vi "DriveWaitForButton.vi"(2 "Parameter String":string, 3 "Reinit":bool) -> (0 "Error Out":errorcluster, 1 "Increment":bool)   [LabVIEW 2019]
doc: "This VI pauses the drive sequencer until the driver presses the \"advance system check\" button on the joystick, the joystick will rumble while waiting for the button."
uses:
  dscommands.vi
  dsdata.vi
  autoninfo.vi
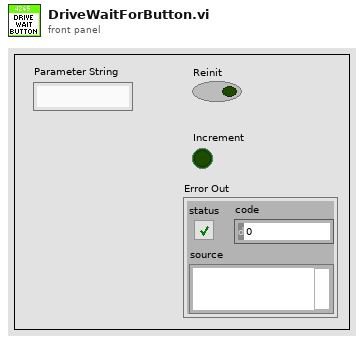
[diagram p1: front panel]
types:
  T1 = enum16{"Center", "North", "NorthWest", "West", "SouthWest", "South", "SouthEast", "East", "NorthEast"}
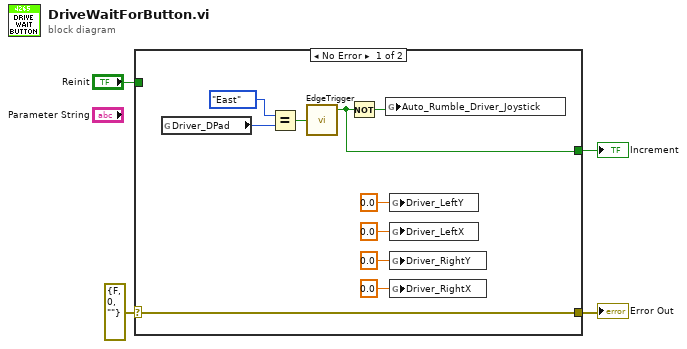
[diagram p0: block diagram]
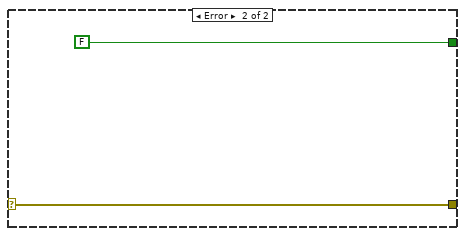
[diagram p2: hidden frame]
diagram:
  n1 = case shown="No Error" errorcluster {"status"=FALSE, "code"=0, "source"=""} ("error IO") {
    selector: errorcluster {"status"=FALSE, "code"=0, "source"=""} ("error IO") -> [w10 w16]
    tunnel: [w5 FALSE] -> w4
    tunnel: "Reinit" -> [_ _]
    tunnel: [w10 w16] -> w2
    frame No Error {
      n2 = global read "dsdata.vi" "Driver_DPad"() -> (w9:T1)
      n3 = Equal?(x=T1."East" ("Driver_DPad"), y=w9) -> (x = y?=w7:bool)
      n4 = call "EdgeTrigger.vi"("Input Signal"=w7) -> ("Rising Edge Trigger"=w5:bool)  [unwired: 2 out]
      n5 = Not(x=w5) -> (.not. x?=w8:bool)
      n6 = global write "autoninfo.vi" "Auto_Rumble_Driver_Joystick"(w8) -> ()
      n7 = global write "dscommands.vi" "Driver_LeftY"(0.0 ("Driver_LeftY")) -> ()
      n8 = global write "dscommands.vi" "Driver_LeftX"(0.0 ("Driver_RightX")) -> ()
      n9 = global write "dscommands.vi" "Driver_RightY"(0.0 ("Driver_RightX")) -> ()
      n10 = global write "dscommands.vi" "Driver_RightX"(0.0 ("Driver_RightX")) -> ()
    }
    frame Error {
    }
  }
  "Increment" <- w4
  "Error Out" <- w2
